vi "Genauigkeit Polynom 2 String.vi"() -> (0 "Format-String Polynom 2 Sting":string="%#.9f", 2 "Genauigkeit für Anzeige":i16=18, 3 "Genauigkeit Polynom 2 String":i16=15)   [LabVIEW 2020, in "Linearisierung v2.lvlib"]
uses:
  Linearisierung v2.lvlib
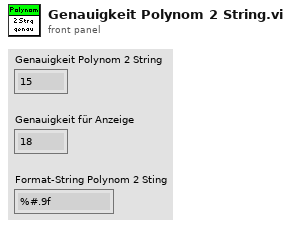
[diagram p1: front panel]
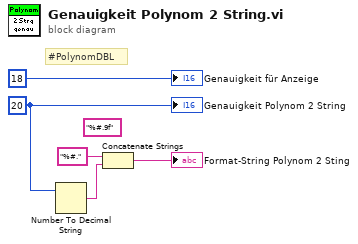
[diagram p0: block diagram]
diagram:
  (unwired) "%#.9f" ("Format-String")
  w5 = i16 20 ("Genauigkeit (6)")
  # "#PolynomDBL"
  n1 = Number To Decimal String(number=w5) -> (decimal integer string=w4:string)  [unwired: 1 in]
  n2 = Concatenate Strings("%#." ("Format-String"), w4) -> (→"Format-String Polynom 2 Sting":string)
  "Genauigkeit Polynom 2 String" <- w5
  "Genauigkeit für Anzeige" <- i16 18 ("Genauigkeit (6)")
